vi "GEA2 HEWH Appliance Data.vi"(0 ".NET Refnum in":refnum<k24>, 1 "LV Program":T5, 2 "GEA2 Event Registration In":refnum<event-registration>, 3 "Disable Electronic Mixing Valve (EMV) List":bool, 4 "Disable Classic GEA2":bool, 5 "error in (no error)":errorcluster, 6 "Enable Diagnostic Data":T2, 7 "#ERDs per message":i32=15, 8 "GEA2?":bool, 9 "Disable ERD A":bool, 11 "Retry Count":i32=5) -> (12 "Converted Data Out":T3 {"CRC" format="%04x"; "Length" format="%02x"; "Command" format="%02x"; "Destination" format="%02x"; "Source" format="%02x"}, 13 "ERD Data Out":T4[](array[typedef]) {"ERD Number" format="%.0x"}, 14 ".NET Refnum out":refnum<k24>, 15 "UnRead ERDs":i32, 16 "GEA2 Event Registration Out":refnum<event-registration>, 17 "HEWH Appliance Data ERD":string[][](array[string]), 19 "error out":errorcluster)   [LabVIEW 2016]
uses:
  type defs/Data Out.ctl
  C:/TechnologyLab/NI-2010/Trunk/Utility/LabVIEW GEA2 Toolkit v1.0.0.0/Appliance.NET/GeaCommunication.dll
  Appliance.NET/GeaCommunication.dll
  Save File/File Setup (Public)/Type Definition/Save File DOE LabView Program.ctl
  type defs/ERD Read Data Out.ctl
  Washer HCC/Washer HCC NEWFI/Type Definitions/HCC Washer Types.ctl
  type defs/Data In.ctl
  GEA2 Commands/HEWH/Type Definitions/GEA2 Commands.ctl
  library/GEA2_Toolkit.lvlib
  Save File/File Setup.lvlib
panel:
  out "Input Data":T1 {"Command" format="%02x"; "Destination" format="%02x"; "Source" format="%02x"}
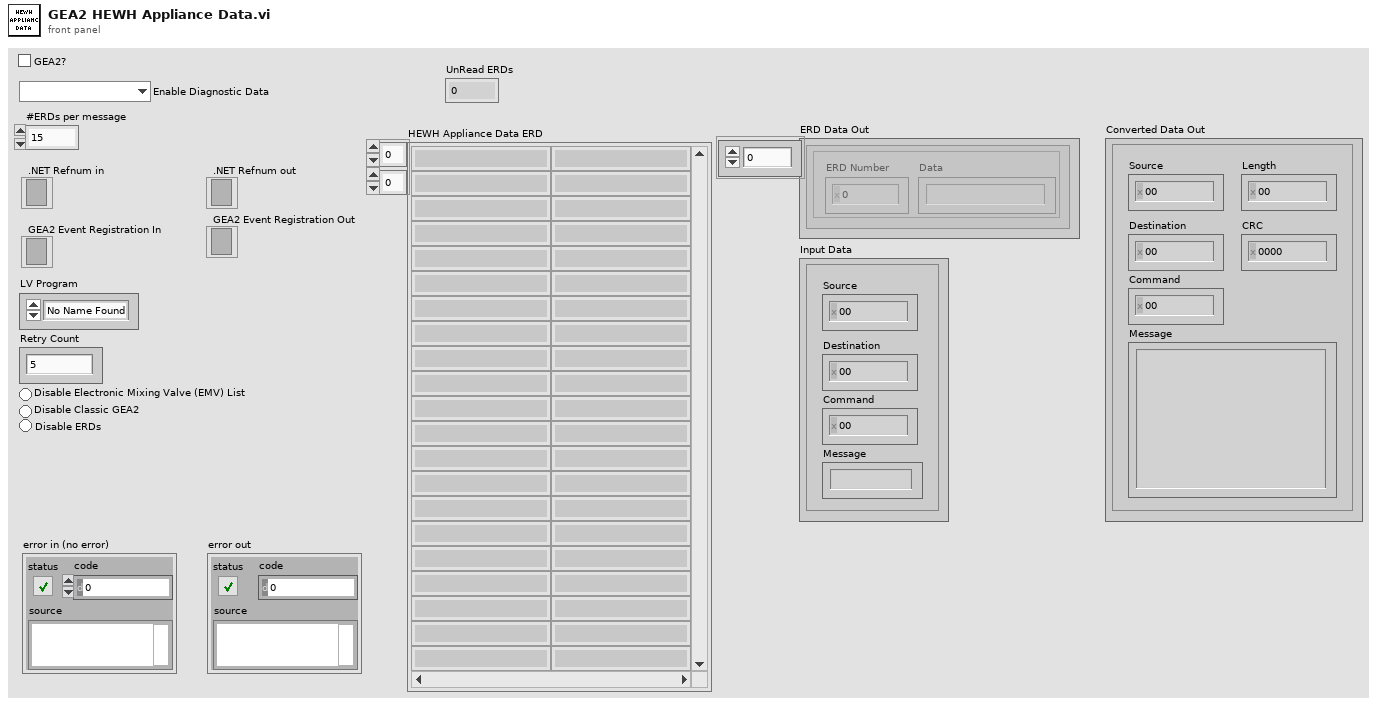
[diagram p1: front panel]
types:
  T1 = typedef "GEA2_Toolkit.lvlib/Data In.ctl" = cluster{"Source":u8, "Destination":u8, "Command":u8, "Message":string}
  T2 = typedef "HCC Washer Types.ctl" = enum16{"", "Viper Washer", "Hawk Washer", "2015 Washer", "2017 Washer"}
  T3 = typedef "GEA2_Toolkit.lvlib/Data Out.ctl" = cluster{"Source":u8, "Destination":u8, "Command":u8, "Length":u8, "CRC":u16, "Message":string}
  T4 = typedef "GEA2_Toolkit.lvlib/ERD Read Data Out.ctl" = cluster{"ERD Number":u16, "Data":string}
  T5 = typedef "File Setup.lvlib/Save File DOE LabView Program.ctl" = enum16{"No Name Found", "DOE Stand", "Dishwasher Kitchen", "Portable Stand", "HEWH", "Dryer", "Dryer WILT", "HCC", "PRAT", "HEWH RLT", "Refrigeration"}
  T6 = typedef "GEA2 Commands.ctl" = enum16{"CMD_CANCEL_EEV_POSITION", "CMD_CLEAR_ENERGY_USAGE_CTRS", "CMD_CLEAR_FAULT_COUNTS", "CMD_CLEAR_OVERRIDE_STATUS", "CMD_COMP_OFF", "CMD_COMP_ON", "CMD_DSM_OVERRIDES", "CMD_EEV_POSITION", "CMD_ENTER_EXIT_FCT_MODE", "CMD_ENTER_FACT_MODE", "CMD_HP_RUN_6MIN", "CMD_INITIATE_REMOTE_DSM_OVERRIDE", "CMD_LE_2_SECONDS", "CMD_REFRESH_SERVICE_TIMEOUTS", "CMD_RESET", "CMD_RESET_FILTER_TIMES", "CMD_RESTORE_EEPROM_DEFAULTS", "CMD_RQST_LED_STATUS", "CMD_SET_AMBIENT_THRESH_1", "CMD_SET_AMBIENT_THRESH_2", "CMD_SET_AMBIENT_THRESH_3", "CMD_SET_CURRENTS", "CMD_SET_EEV_DRIVE_LINES", "CMD_SET_EEV_STOP_POSITION", "CMD_SET_LEDS", "CMD_SET_MODEL_NUMBER", "CMD_SET_PID_I_DENOM_OVER_THR", "CMD_SET_PID_I_DENOM_UNDER_THR", "CMD_SET_PID_LOW_SH_TARGET", "CMD_SET_PID_MID_SH_TARGET", "CMD_SET_PID_P_DENOMINATOR", "CMD_SET_SERIAL_NUMBER", "CMD_SET_START_POS_OVER_THR", "CMD_SET_START_POS_UNDER_THR", "CMD_TOGGLE_FAN", "CMD_TOGGLE_LE_SERV", "CMD_TOGGLE_SERVICE_MODE", "CMD_TOGGLE_UE_SERV", "CMD_TURN_ON_OFF_DLB", "CMD_UE_2_SECONDS", "CMD_UPDATE_DSM_LEVEL", "CMD_UPDATE_MODE", "CMD_WRITE_SETPOINTS", "REQ_READ_KEY_STATUS", "REQ_SYSTEM_MODE", "RQST_CURRENT_PID_SH_TARGET", "RQST_DATA_FROM_DATA_FLASH", "RQST_DATA_FROM_MEMORY", "RQST_DSM_OVERRIDE_STATUS", "RQST_HEM_KWH_DATA", "RQST_HYPERTERM_OUTPUT_DATA", "RQST_IDLB_RESISTANCE", "RQST_MODEL_NUMBER", "RQST_MODEL_SELECT_AD_VALUE", "RQST_OTHER_FAULT_COUNTS", "RQST_OVERRIDE_STATUS", "RQST_PID_PARAMETERS", "RQST_READ_PERSONALITY", "RQST_SERIAL_NUMBER", "RQST_SERVICE_ERROR_CODES", "RQST_Software_Version", "RQST_SS_FAULT_COUNTS", "RQST_STATUS_QUERY", "RQST_STD_ELEC_RANGE", "RQST_SUPPORTED_MODES", "RQST_T2_RESISTANCE", "RQST_T3B_RESISTANCE", "RQST_T4_RESISTANCE", "RQST_T5_RESISTANCE", "RQST_TEMP_RANGE", "RQST_VACATION_RANGE", "RQST_WATER_CAPACITY"}
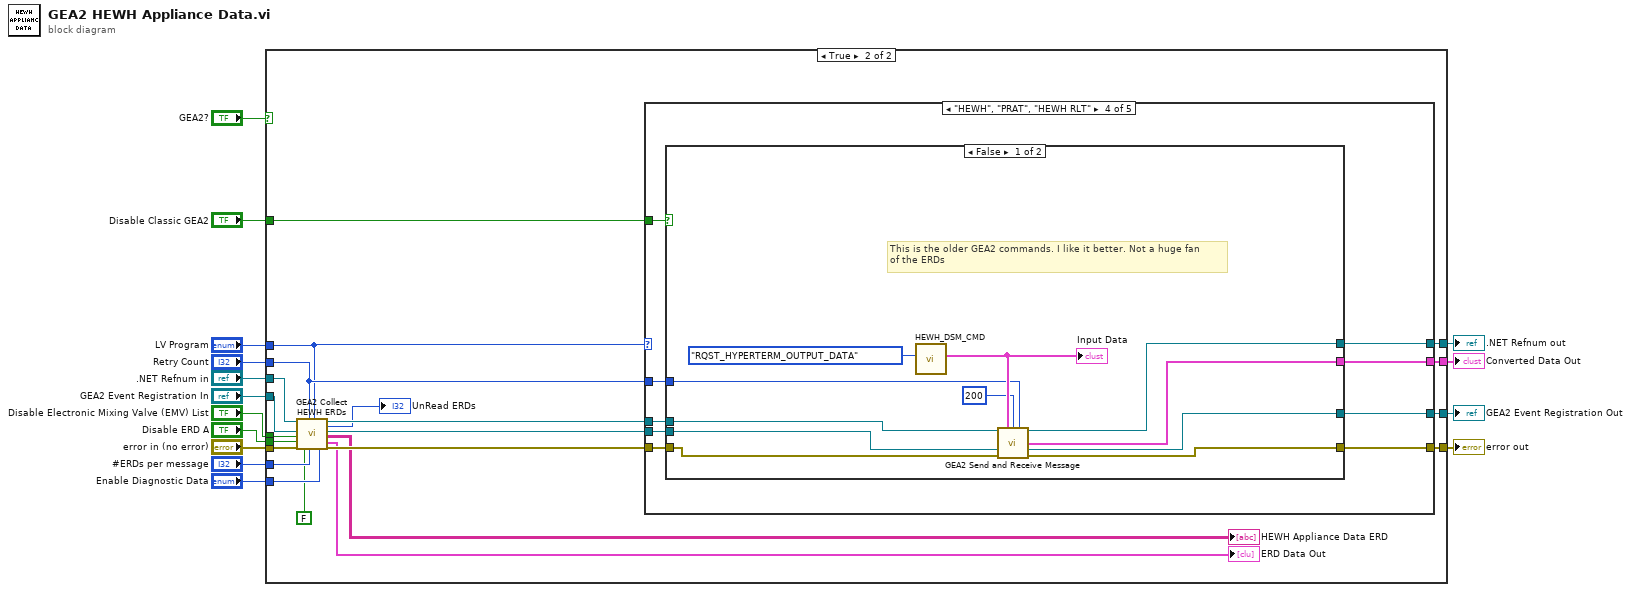
[diagram p0: block diagram]
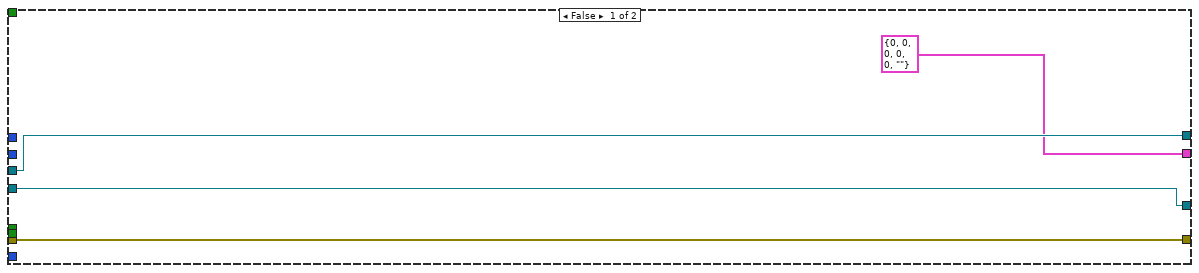
[diagram p2: hidden frame]
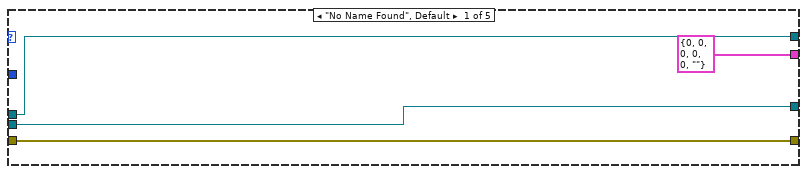
[diagram p3: hidden frame]
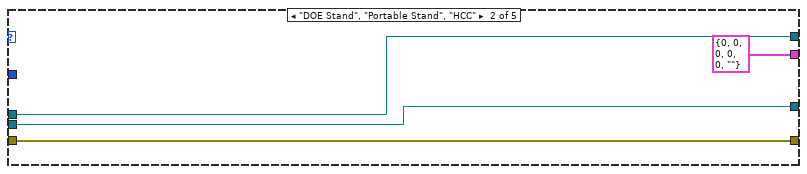
[diagram p4: hidden frame]
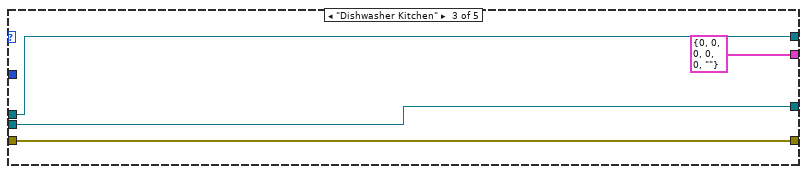
[diagram p5: hidden frame]
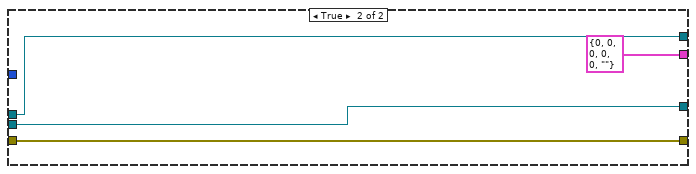
[diagram p6: hidden frame]
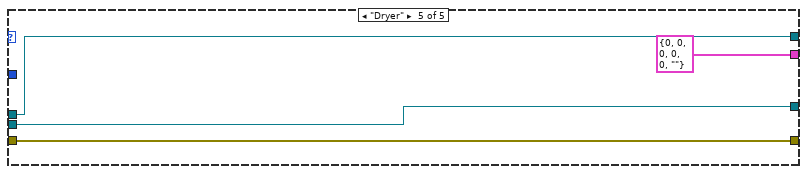
[diagram p7: hidden frame]
diagram:
  n1 = case shown="True" "GEA2?" {
    tunnel: "GEA2 Event Registration In" -> [w18 w39]
    tunnel: ".NET Refnum in" -> [w19 w37]
    tunnel: "Disable Electronic Mixing Valve (EMV) List" -> [_ w36]
    tunnel: "error in (no error)" -> [w17 w34]
    tunnel: [w19 w33] -> w11
    tunnel: [w18 w32] -> w10
    tunnel: [w17 w31] -> w9
    tunnel: "Disable ERD A" -> [_ w30]
    tunnel: "Retry Count" -> [_ w29]
    tunnel: "LV Program" -> [_ w28]
    tunnel: "Disable Classic GEA2" -> [_ w27]
    tunnel: "#ERDs per message" -> [_ w25]
    tunnel: [T3 {"Source"=0, "Destination"=0, "Command"=0, "Length"=0, "CRC"=0, "Message"=""} ("Converted Data Out") w24] -> w3
    tunnel: "Enable Diagnostic Data" -> [_ w22]
    frame False {
    }
    frame True {
      n2 = call "GEA2 Collect HEWH ERDs.vi"(".NET Refnum in"=w37, "GEA2 Event Registration In"=w39, "Disable Electronic Mixing Valve (EMV) List"=w36, "Disable ERD (Main)"=w30, "error in (no error)"=w34, "Disable ERD Filter"=FALSE, "Retry Count"=w29, "#ERDs per message"=w25, "LV Program"=w28, "Enable Diagnostic Data"=w22) -> ("ERD Data Out"=→"ERD Data Out":T4[], ".NET Refnum out"=w38:refnum<k24>, "UnRead ERDs"=→"UnRead ERDs":i32, "GEA2 Event Registration Out"=w40:refnum<event-registration>, "ERD Array"=→"HEWH Appliance Data ERD":string[][], "error out"=w35:errorcluster)  [unwired: 4 in]
      n3 = case shown="\"HEWH\", \"PRAT\", \"HEWH RLT\"" w28 {
        tunnel: w40 -> [w43 w48 w51 w61 w79]
        tunnel: w38 -> [w44 w47 w52 w60 w80]
        tunnel: w35 -> [w42 w46 w50 w59 w78]
        tunnel: [w44 w47 w52 w58 w80] -> w33
        tunnel: [w43 w48 w51 w57 w79] -> w32
        tunnel: [w42 w46 w50 w56 w78] -> w31
        tunnel: w29 -> [_ _ _ w55 _]
        tunnel: w27 -> [_ _ _ w54 _]
        tunnel: [T3 {"Source"=0, "Destination"=0, "Command"=0, "Length"=0, "CRC"=0, "Message"=""} ("Converted Data Out") T3 {"Source"=0, "Destination"=0, "Command"=0, "Length"=0, "CRC"=0, "Message"=""} ("Converted Data Out") T3 {"Source"=0, "Destination"=0, "Command"=0, "Length"=0, "CRC"=0, "Message"=""} ("Converted Data Out") w53 T3 {"Source"=0, "Destination"=0, "Command"=0, "Length"=0, "CRC"=0, "Message"=""} ("Converted Data Out")] -> w24
        frame "No Name Found", Default {
        }
        frame "DOE Stand", "Portable Stand", "HCC" {
        }
        frame "Dishwasher Kitchen" {
        }
        frame "HEWH", "PRAT", "HEWH RLT" {
          n4 = case shown="False" w54 {
            tunnel: w61 -> [w72 w75]
            tunnel: w60 -> [w71 w76]
            tunnel: w59 -> [w69 w74]
            tunnel: [w67 w76] -> w58
            tunnel: [w63 w75] -> w57
            tunnel: [w64 w74] -> w56
            tunnel: w55 -> [w66 _]
            tunnel: [w62 T3 {"Source"=0, "Destination"=0, "Command"=0, "Length"=0, "CRC"=0, "Message"=""} ("Converted Data Out")] -> w53
            frame False {
              # "This is the older GEA2 commands. I like it better. Not a huge fan\nof the ERDs"
              n5 = call "HEWH_DSM_CMD.vi"("GEA2 Commands and Requests"=GEA2_Commands."RQST_HYPERTERM_OUTPUT_DATA") -> ("Input Data"=w68:T1)  [unwired: 8 in, 1 out]
              "Input Data" <- w68
              n6 = call "GEA2 Send and Receive Message.vi"("GEA2 Reference In"=w71, "Input Data"=w68, "Read Timeout (ms)"=u32 200, "# of Retries"=w66, "GEA2 Event Registration"=w72, "Error In"=w69) -> ("GEA2 Reference Out"=w67:refnum<k24>, "Converted Data Out"=w62:T3, "Event Registration Out"=w63:refnum<event-registration>, "Error Out"=w64:errorcluster)  [unwired: 4 in, 2 out]
            }
            frame True {
            }
          }
        }
        frame "Dryer" {
        }
      }
    }
  }
  "error out" <- w9
  ".NET Refnum out" <- w11
  "GEA2 Event Registration Out" <- w10
  "Converted Data Out" <- w3
